vi "Get Method Call Event Ref.vi"(8 "error in (no error)":errorcluster, 11 "JKI_Python_Server in":refnum<class "Server.lvclass">) -> (0 "error out":errorcluster, 1 "Methods (VEnum)":variant, 2 "Python Method Call":refnum<user-event>, 3 "JKI_Python_Server out":refnum<class "Server.lvclass">)   [LabVIEW 2013, in "JKI_Python_Bridge_for_LV.lvlib" / "Server.lvclass"]
uses:
  Server.lvclass
  Call/Call.lvclass
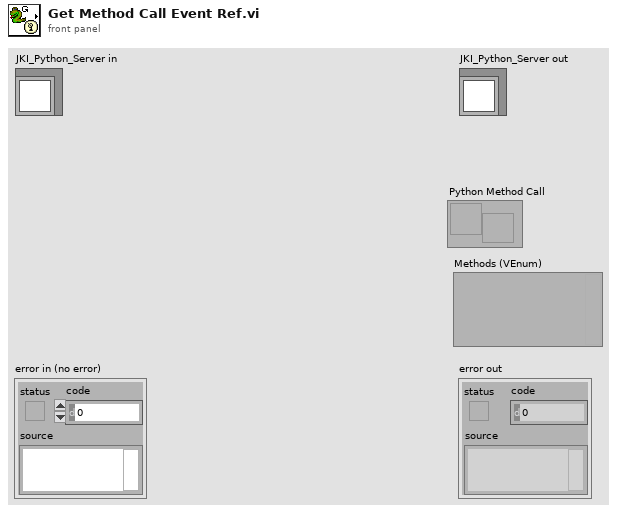
[diagram p1: front panel]
types:
  T1 = typedef "JKI_Python_Bridge_for_LV.lvlib/Server.lvclass/Class Private Data - Cluster.ctl" = cluster{"TCP Server RefNum":T2, "TCP port (50007)":u16, "max connections (0: no limit)":u32, "net address (0: Listen on All Adaptors)":u32, "Nodes":T3[], "Public Events":T4}
  T2 = typedef "TCP Server Object RefNum__jki_lib_tcp_server.ctl" = refnum<k1>
  T3 = typedef "JKI_Python_Bridge_for_LV.lvlib/Server.lvclass/Python Node.ctl" = cluster{"Name":string, "Python Method Call":refnum<user-event>, "Node":refnum<class "Node.lvclass">}
  T4 = typedef "JKI_Python_Bridge_for_LV.lvlib/Server.lvclass/Public Events - Cluster.ctl" = cluster{"Stop Nodes":refnum<user-event>}
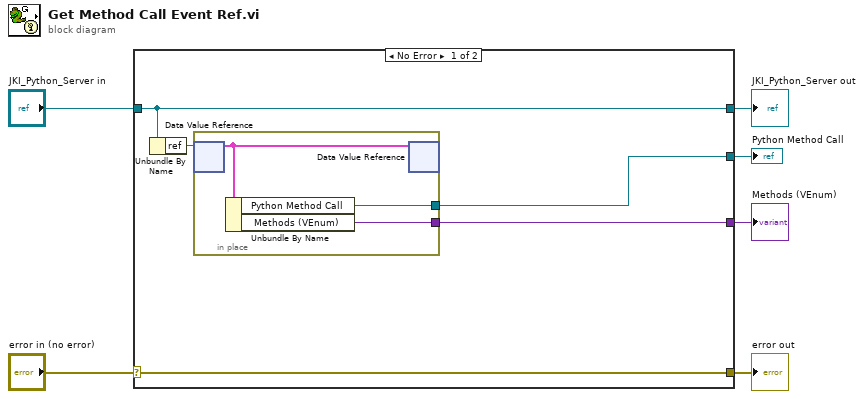
[diagram p0: block diagram]
diagram:
  n1 = case shown="No Error" "error in (no error)" {
    selector: "error in (no error)" -> [w8 w16]
    tunnel: [w8 w16] -> w5
    tunnel: [w11 w15] -> w3
    tunnel: "JKI_Python_Server in" -> [w11 w15]
    tunnel: [w9 _] -> w2
    tunnel: [w7 _] -> w1
    frame No Error {
      n2 = Unbundle By Name(w11) -> ("ref"=w10:refnum<data-value>)
      n3 = in-place {
        in-place-border: [w13] -> w9
        in-place-border: [w12] -> w7
        n4 = in-place-dvr #1(w10) -> (w14:T1)  [unwired: 1 out]
        n5 = Unbundle By Name(w14) -> ("Python Method Call"=w13:refnum<user-event>, "Methods (VEnum)"=w12:variant)
        n6 = in-place-dvr #1(w14) -> ()  [unwired: 2 out]
      }
    }
    frame Error {
    }
  }
  "error out" <- w5
  "JKI_Python_Server out" <- w3
  "Python Method Call" <- w2
  "Methods (VEnum)" <- w1
